vi "setHeater.vi"(6 "Channel":i32, 8 "error in (no error)":errorcluster, 10 "Current (mA)":dbl, 11 "Instrument.TC in":refnum<class "Inst.TC.lvclass">) -> (0 "error out":errorcluster, 3 "Instrument.TC out":refnum<class "Inst.TC.lvclass">)   [LabVIEW 2019, in "Inst.TC.lvclass"]
uses:
  Inst.TC.lvclass
  <userlib>/LevyLab/Instrument Framework/Instrument Types/Cryostat/Instrument.Cryostat.lvclass
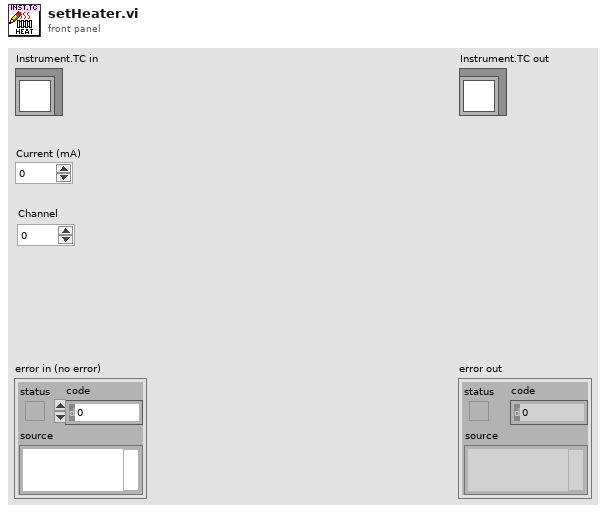
[diagram p1: front panel]
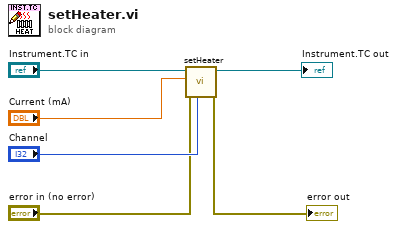
[diagram p0: block diagram]
diagram:
  n1 = call-parent "setHeater.vi"("Channel"="Channel", "error in (no error)"="error in (no error)", "Current (A)"="Current (mA)", "Instrument.Cryostat in"="Instrument.TC in") -> ("error out"=→"error out":errorcluster, "Instrument.Cryostat out"=→"Instrument.TC out":refnum<class "Inst.TC.lvclass">)  [unwired: 6 in]
